vi "match address and function code.vi"(0 "Address":string, 2 "Received Address":string, 3 "Received Function Code":string, 9 "Function Code":string, 11 "NewCmd":bool) -> (4 "Address?":bool, 10 "FCode?":bool)   [LabVIEW 2014, in "HPCNC.lvlib"]
uses:
  HPCNC.lvlib
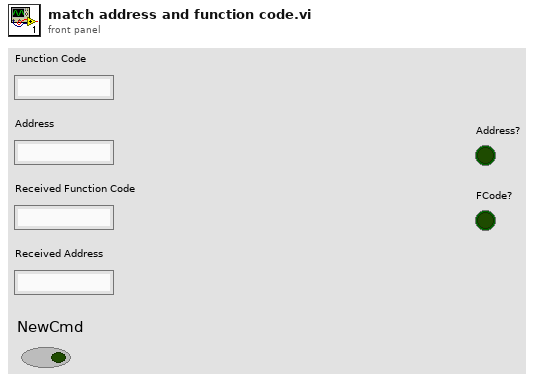
[diagram p1: front panel]
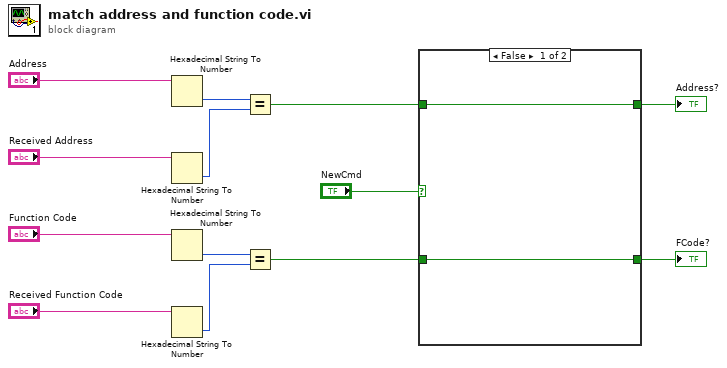
[diagram p0: block diagram]
diagram:
  n1 = Hexadecimal String To Number(string="Address") -> (number=w9:u32)  [unwired: 2 in, 1 out]
  n2 = Hexadecimal String To Number(string="Received Address") -> (number=w8:u32)  [unwired: 2 in, 1 out]
  n3 = Hexadecimal String To Number(string="Function Code") -> (number=w7:u32)  [unwired: 2 in, 1 out]
  n4 = Hexadecimal String To Number(string="Received Function Code") -> (number=w6:u32)  [unwired: 2 in, 1 out]
  n5 = Equal?(x=w9, y=w8) -> (x = y?=w3:bool)
  n6 = Equal?(x=w7, y=w6) -> (x = y?=w1:bool)
  n7 = case shown="False" "NewCmd" {
    selector: "NewCmd" -> [_ w16]
    tunnel: [w15 w16] -> w4
    tunnel: w3 -> [w15 _]
    tunnel: [w14 w16] -> w2
    tunnel: w1 -> [w14 _]
    frame False {
    }
    frame True {
    }
  }
  "Address?" <- w4
  "FCode?" <- w2
